vi "Search Reg Exp in Multiline String.vi"(2 "Regular Expression":string, 3 "Multiline String In":string) -> (0 "Lines Contains Reg EXP":i32[](array[numeric]), 1 "Multiline String Out":string)   [LabVIEW 2019]
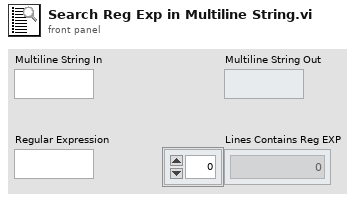
[diagram p1: front panel]
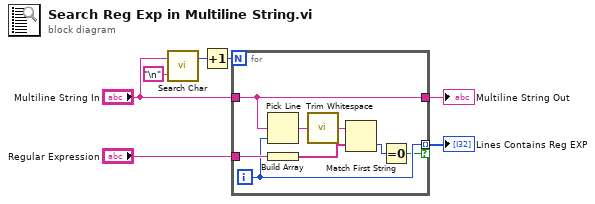
[diagram p0: block diagram]
diagram:
  n1 = call "Search Char.vi"("Search Char"="\n", "Multiline String"="Multiline String In") -> ("Number of Char Found"=w6:i32)  [unwired: 1 out]
  n2 = Increment(x=w6) -> (x+1=w5:i32)
  n3 = for {
    N: w5 -> [_]
    tunnel: "Multiline String In" -> [w13]
    tunnel: "Regular Expression" -> [w15]
    tunnel: [w9] -> w2 mode=indexing if=w8
    tunnel: [w13] -> w1
    i -> [w9]
    n4 = Pick Line(multi-line string=w13, line index=w9) -> (output string=w12:string)  [unwired: 1 in]
    n5 = Build Array(w15) -> (w14:string[])
    n6 = call <vilib>:"Trim Whitespace.vi"("string"=w12) -> ("trimmed string"=w11:string)  [unwired: 1 in]
    n7 = Match First String(2:w14, 3:w11) -> (0:w10:i32)  [unwired: 1 out]
    n8 = Equal To 0?(x=w10) -> (x = 0?=w8:bool)
  }
  "Multiline String Out" <- w1
  "Lines Contains Reg EXP" <- w2
